vi "32ScanBarcodeJW - old.vi"(4 "no check?":bool, 6 "条码长度":i32=6, 7 "总数":i32=6) -> (0 "电子表格字符串":string, 1 "Barcodes out":string[](array[string]), 2 "canceled":bool, 3 "PF":bool[](array[boolean]))   [LabVIEW 2018]
uses:
  Global.vi
panel:
  in  "重置":bool
  out "长度":i32
  out "数组":string[](array[string])
  out "Length 2":i32
  in  "Barcode 32":string
  in  "Barcode31":string
  in  "Barcode 30":string
  in  "Barcode 29":string
  in  "Barcode 28":string
  in  "Barcode 27":string
  in  "Barcode 26":string
  in  "Barcode 25":string
  in  "Barcode 24":string
  in  "Barcode23":string
  in  "Barcode22":string
  in  "Barcode 21":string
  in  "Barcode 20":string
  in  "Barcode 19":string
  in  "Barcode 18":string
  in  "Barcode17":string
  in  "Barcode 16":string
  in  "Barcode 15":string
  in  "Barcode 14":string
  in  "Barcode 13":string
  in  "Barcode 12":string
  in  "Barcode 11":string
  in  "Barcode 10":string
  in  "Barcode 9":string
  in  "Barcode 8":string
  in  "Barcode 7":string
  in  "Barcode 6":string
  in  "Barcode 5":string
  in  "Barcode 4":string
  in  "Barcode 3":string
  in  "Barcode 2":string
  in  "Barcode 1":string
  out "barcode refrencesd":refnum<vi>[](array[refnum])
  in  "esc":bool
  in  "OK":bool
  # "请使用扫描枪扫描条码或二维码!放弃请按\"ESC\"键!"
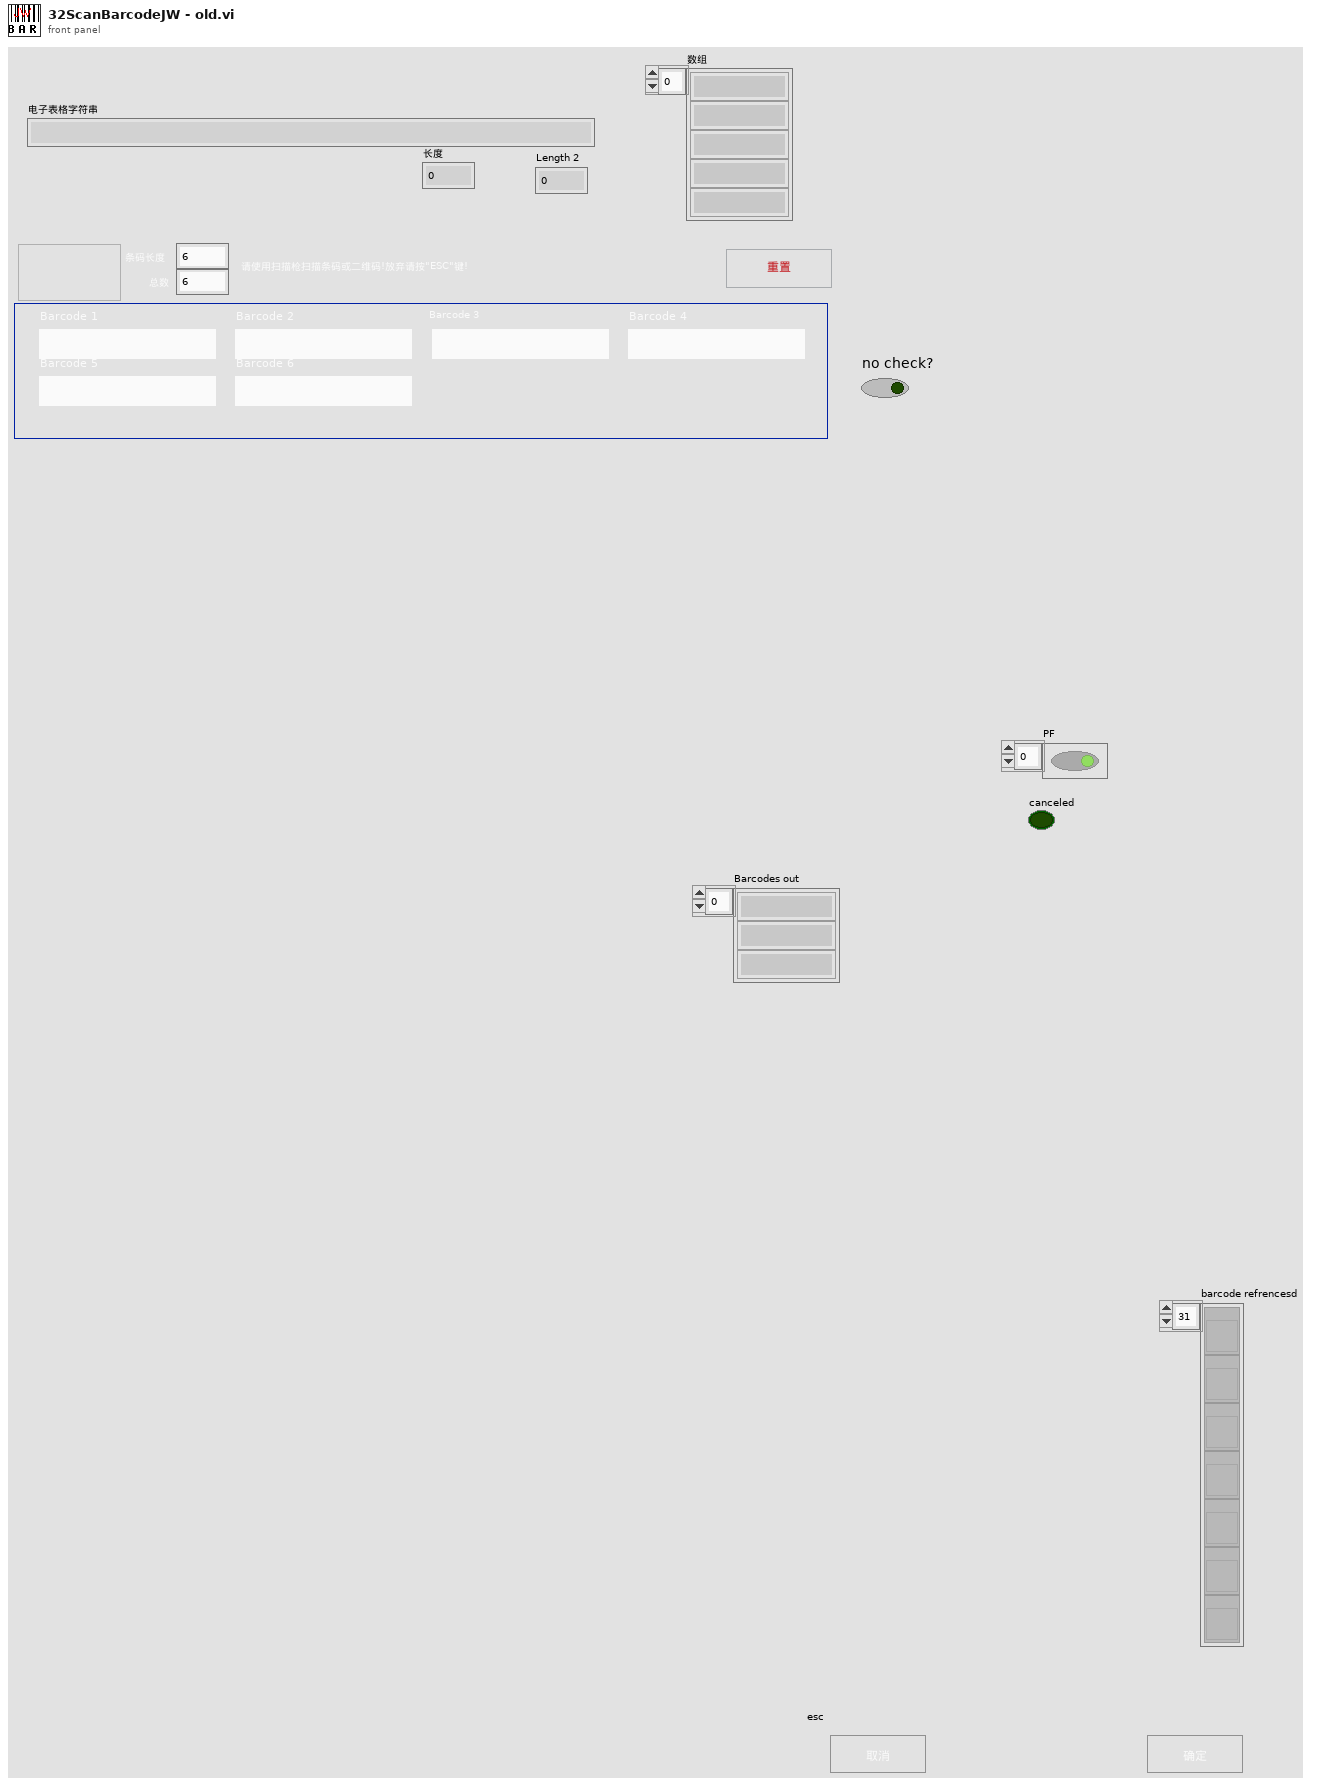
[diagram p1: front panel]
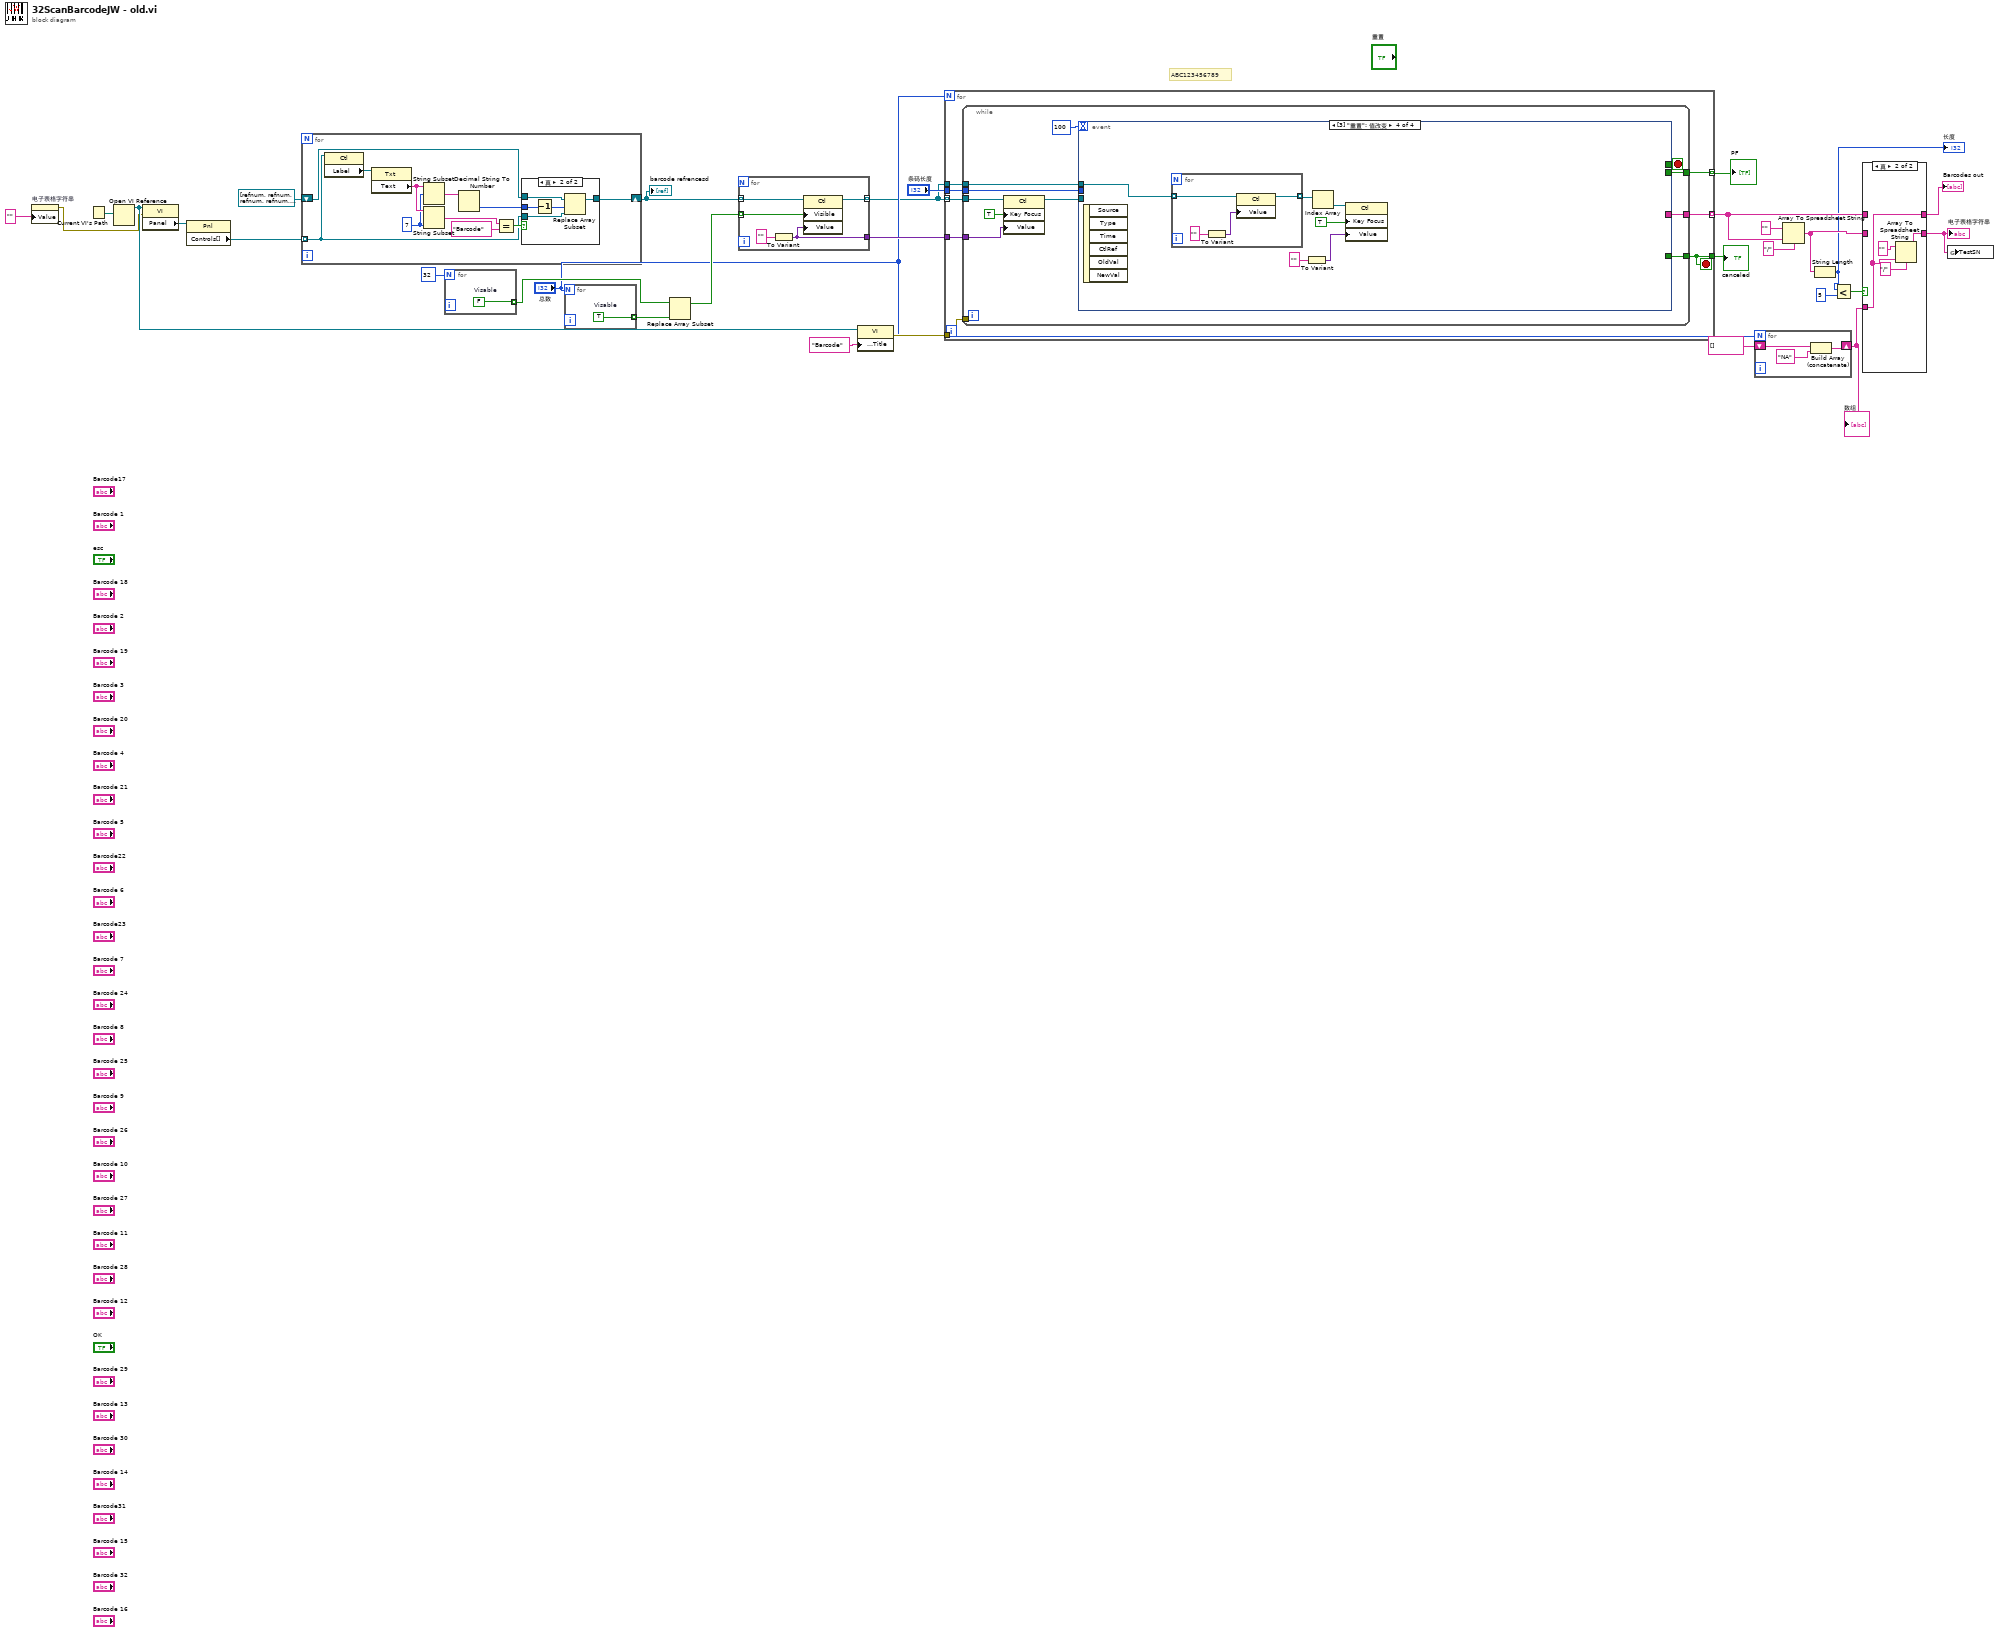
[diagram p0: block diagram]
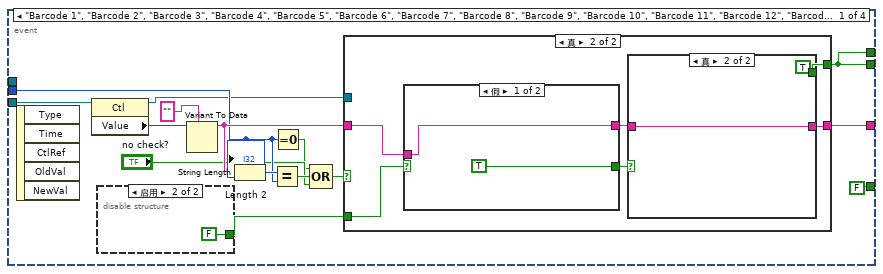
[diagram p3: hidden frame]
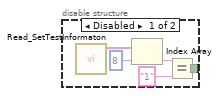
[diagram p4: hidden frame]
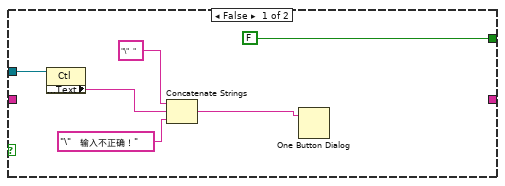
[diagram p5: hidden frame]
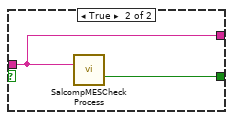
[diagram p6: hidden frame]
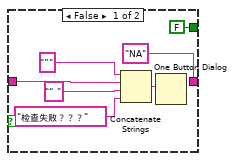
[diagram p7: hidden frame]
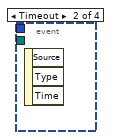
[diagram p8: hidden frame]
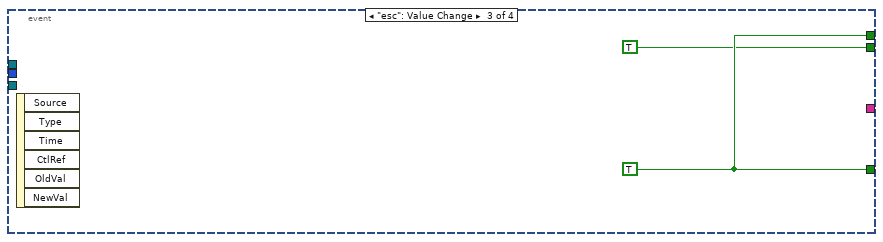
[diagram p9: hidden frame]
diagram:
  # "ABC123456789"
  n1 = property on="电子表格字符串" class="Str"("Value"="") -> (error out=w5:errorcluster)  [unwired: 2 in, 1 out]
  n2 = Current VI's Path() -> (path=w31:path)
  n3 = Open VI Reference(vi path=w31) -> (vi reference=w28:refnum<vi>)  [unwired: 2 in, 4 out]
  n4 = property class="VI"(reference=w28, error in=w5) -> ("Panel"=w27:refnum<vi>)  [unwired: 2 out]
  n5 = property class="Pnl"(reference=w27) -> ("Controls[]"=w26:refnum<vi>[])  [unwired: 1 in, 2 out]
  n6 = for {
    tunnel: w26 -> [w32] mode=indexing
    shift-right: [w41] -> w25
    shift-left: refnum<vi>[] [refnum, refnum, refnum, refnum, refnum, refnum, refnum, refnum, refnum, refnum, refnum, refnum, refnum, refnum, refnum, refnum, refnum, refnum, refnum, refnum, refnum, refnum, refnum, refnum, refnum, refnum, refnum, refnum, refnum, refnum, refnum, refnum] ("barcode refrencesd 2") -> [w42]
    w35 = 7 ("长度（剩余）")
    n7 = property class="Ctl"(reference=w32) -> ("Label"=w40:refnum<vi>)  [unwired: 1 in, 2 out]
    n8 = property class="Txt"(reference=w40) -> ("Text"=w36:string)  [unwired: 1 in, 2 out]
    n9 = String Subset(string=w36, offset (0)=w35) -> (substring=w34:string)  [unwired: 1 out]
    n10 = String Subset(string=w36, length (rest)=w35) -> (substring=w38:string)  [unwired: 1 out]
    n11 = Decimal String To Number(string=w34) -> (number=w33:i32)  [unwired: 3 out]
    n12 = Equal?(x=w38, y="Barcode") -> (x = y?=w37:bool)
    n13 = case shown="真" w37 {
      tunnel: w42 -> [w43 w48]
      tunnel: [w43 w47] -> w41
      tunnel: w33 -> [_ w46]
      tunnel: w32 -> [_ w44]
      frame False {
      }
      frame True {
        n14 = Decrement(x=w46) -> (x-1=w45:i32)
        n15 = Replace Array Subset(array=w48, new element=w44, index=w45) -> (w47:refnum<vi>[])
      }
    }
  }
  "barcode refrencesd" <- w25
  n16 = for {
    N: 32 -> [_]
    tunnel: [w49] -> w24 mode=indexing
    w49 = FALSE  # Visable
  }
  n17 = for {
    N: "总数" -> [_]
    tunnel: [w50] -> w15 mode=indexing
    w50 = TRUE  # Visable
  }
  n18 = Replace Array Subset(array=w24, new element=w15) -> (w23:bool[])  [unwired: 1 in]
  n19 = for {
    tunnel: w25 -> [w55] mode=indexing
    tunnel: w23 -> [w54] mode=indexing
    tunnel: [w52] -> w1 mode=indexing
    tunnel: [w51] -> w19
    n20 = To Variant(anything="") -> (Variant=w51:variant)
    n21 = property class="Ctl"(reference=w55, "Visible"=w54, "Value"=w51) -> (reference out=w52:refnum<vi>)  [unwired: 1 in, 1 out]
  }
  n22 = property class="VI"(reference=w28, "Front Panel.Title"="Barcode" ("前面板窗口:标题")) -> (error out=w30:errorcluster)  [unwired: 1 in, 1 out]
  n23 = for {
    N: "总数" -> [_]
    tunnel: w30 -> [w63]
    tunnel: [w62] -> w11 mode=indexing
    tunnel: [w61] -> w20 mode=indexing
    tunnel: w1 -> [w60] mode=indexing
    tunnel: "条码长度" -> [w59]
    tunnel: w19 -> [w58]
    tunnel: [w57] -> w18
    tunnel: w1 -> [w56]
    stop <- w57 stop-if-true
    n24 = while {
      tunnel: [w70] -> w61
      tunnel: [w74] -> w62
      tunnel: w63 -> [_]
      tunnel: w60 -> [w66]
      tunnel: w59 -> [w71]
      tunnel: w58 -> [w65]
      tunnel: [w67] -> w57
      tunnel: w56 -> [w64]
      stop <- w68 stop-if-true
      n25 = property class="Ctl"(reference=w66, "Key Focus"=TRUE ("键选中"), "Value"=w65) -> (reference out=w72:refnum<vi>)  [unwired: 1 in, 1 out]
      n26 = event shown="[3] \"重置\": 值改变" {
        selector: _ -> [_ _ _ _]
        dyn-events: _ -> [_ _ _ _]
        timeout: 100 -> [_ _ _ _]
        tunnel: [w88 _ _ _] -> w74
        tunnel: w72 -> [w87 _ _ _]
        tunnel: w71 -> [w83 _ _ _]
        tunnel: [w82 _ w122 _] -> w68
        tunnel: [w82 _ TRUE _] -> w70
        tunnel: [FALSE _ w122 _] -> w67
        tunnel: w64 -> [_ _ _ w128]
        event "Barcode 1", "Barcode 2", "Barcode 3", "Barcode 4", "Barcode 5", "Barcode 6", "Barcode 7", "Barcode 8", "Barcode 9", "Barcode 10", "Barcode 11", "Barcode 12", "Barcode 13", "Barcode 14", "Barcode 15", "Barcode 16", "Barcode17", "Barcode 18", "Barcode 19", "Barcode 20", "Barcode 21", "Barcode22", "Barcode23", "Barcode 24", "Barcode 26", "Barcode 25", "Barcode 27", "Barcode 28", "Barcode 29", "Barcode 30", "Barcode31", "Barcode 32": Value Change {
          n27 = event-data() -> ()  [unwired: 6 out]
          n28 = property class="Ctl"(reference=w87) -> (reference out=w77:refnum<vi>, "Value"=w86:variant)  [unwired: 1 in, 1 out]
          n29 = disable-structure shown="启用" {
            disable-tunnel: [w90 FALSE] -> w75
            frame Disabled {
              n30 = call "Read_SetTestInformaton.vi"() -> ("数组 2"=w94:string[])  [unwired: 8 in, 3 out]
              n31 = Index Array(array=w94, index=8 ("索引")) -> (element=w93:string)
              n32 = Equal?(x=w93, y="1") -> (x = y?=w90:bool)
            }
            frame Enabled {
            }
          }
          n33 = Variant To Data(type="", Variant=w86) -> (data=w84:string)  [unwired: 1 in, 1 out]
          n34 = String Length(string=w84) -> (length=w89:i32)
          n35 = Equal?(x=w89, y=w83) -> (x = y?=w81:bool)
          n36 = Equal To 0?(x=w83) -> (x = 0?=w78:bool)
          n37 = Compound Arithmetic op=OR(w78, w81, "no check?") -> (w80:bool)
          n38 = case shown="真" w80 {
            tunnel: [FALSE w107] -> w82
            tunnel: w84 -> [_ w105]
            tunnel: [_ w102] -> w88
            tunnel: w77 -> [w100 _]
            tunnel: w75 -> [_ w104]
            frame False {
              n39 = property class="Ctl"(reference=w100) -> ("Label.Text"=w99:string)  [unwired: 1 in, 2 out]
              n40 = Concatenate Strings("\"  " ("消息"), w99, "\"   输入不正确！" ("消息")) -> (w98:string)
              n41 = One Button Dialog(message=w98) -> ()  [unwired: 2 out]
            }
            frame True {
              n42 = case shown="假" w104 {
                tunnel: [TRUE ("CheckRouteForSerialNumber") w111] -> w106
                tunnel: w105 -> [w108 w110]
                tunnel: [w108 w110] -> w103
                frame False {
                }
                frame True {
                  n43 = call "SalcompMESCheck Process.vi"("SN"=w110) -> ("CheckRouteForSerialNumber"=w111:bool)  [unwired: 12 in, 2 out]
                }
              }
              n44 = case shown="真" w106 {
                tunnel: [FALSE TRUE] -> w107
                tunnel: w103 -> [w114 w119]
                tunnel: ["NA" w119] -> w102
                frame False {
                  n45 = Concatenate Strings("”", w114, "“ ", "检查失败？？？" ("消息")) -> (w117:string)
                  n46 = One Button Dialog(message=w117) -> ()  [unwired: 1 in, 1 out]
                }
                frame True {
                }
              }
            }
          }
          "Length 2" <- w83
        }
        event Timeout {
          n47 = event-data() -> ()  [unwired: 4 out]
        }
        event "esc": Value Change {
          w122 = TRUE
          n48 = event-data() -> ()  [unwired: 7 out]
        }
        event "重置": Value Change {
          n49 = event-data() -> ()  [unwired: 7 out]
          n50 = for {
            tunnel: w128 -> [w132] mode=indexing
            tunnel: [w130] -> w127 mode=indexing
            n51 = To Variant(anything="") -> (Variant=w129:variant)
            n52 = property class="Ctl"(reference=w132, "Value"=w129) -> (reference out=w130:refnum<vi>)  [unwired: 1 in, 1 out]
          }
          n53 = To Variant(anything="") -> (Variant=w123:variant)
          n54 = Index Array(array=w127) -> (element=w126:refnum<vi>)  [unwired: 1 in]
          n55 = property class="Ctl"(reference=w126, "Key Focus"=TRUE ("键选中"), "Value"=w123) -> ()  [unwired: 1 in, 2 out]
        }
      }
    }
  }
  "PF" <- w20
  "canceled" <- w18
  n56 = for {
    N: "总数" -> [_]
    shift-right: [w133] -> w13
    shift-left: string[] [] -> [w134]
    n57 = Build Array (concatenate)(w134, "NA") -> (w133:string[])
  }
  "数组" <- w13
  n58 = Array To Spreadsheet String(delimiter (Tab)="/" ("分隔符(Tab)"), array=w11, 3:"" ("格式字符串")) -> (spreadsheet string=w9:string)
  n59 = String Length(string=w9) -> (length=w8:i32)
  "长度" <- w8
  n60 = Less?(x=w8, y=5) -> (x < y?=w10:bool)
  n61 = case shown="真" w10 {
    tunnel: [w137 w139] -> w2
    tunnel: w9 -> [w137 _]
    tunnel: w13 -> [_ w138]
    tunnel: [w136 w138] -> w12
    tunnel: w11 -> [w136 _]
    frame False {
    }
    frame True {
      n62 = Array To Spreadsheet String(delimiter (Tab)="/" ("分隔符(Tab)"), array=w138, 3:"" ("格式字符串")) -> (spreadsheet string=w139:string)
    }
  }
  "Barcodes out" <- w12
  "电子表格字符串" <- w2
  n63 = global write "Global.vi" "TestSN"(w2) -> ()
